vi "iClassLoader.vi"() -> (0 "iClassLoader":refnum<class "iClassLoader.lvclass">)   [LabVIEW 2020, in "ClassLoader_VIMs.lvlib"]
uses:
  ClassLoader_VIMs.lvlib
  iClassLoader.lvclass
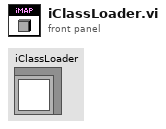
[diagram p1: front panel]
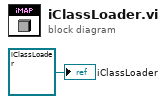
[diagram p0: block diagram]
diagram:
  "iClassLoader" <- refnum<class "iClassLoader.lvclass"> refnum ("ClassLoader.lvlib:iClassLoader.lvclass")
